vi "Write Plot Data.vi"(10 "Plot Data":cluster{dbl[], dbl[]}[](array[cluster]), 11 "MCCW ACLR in":refnum<class "MCCW ACLR.lvclass">) -> (3 "MCCW ACLR out":refnum<class "MCCW ACLR.lvclass">)   [LabVIEW 2020, in "MCCW ACLR.lvclass"]
uses:
  MCCW ACLR.lvclass
  MCCW ACLR.lvclass/MCCW ACLR.ctl
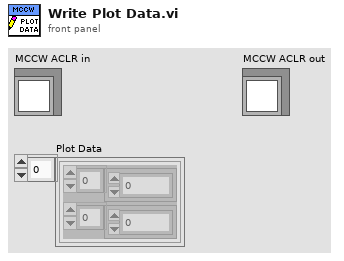
[diagram p1: front panel]
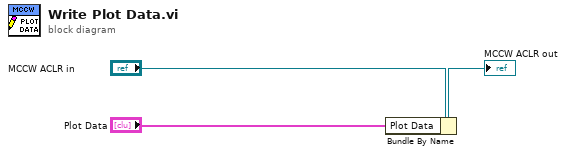
[diagram p0: block diagram]
diagram:
  n1 = Bundle By Name(cluster="MCCW ACLR in", "Plot Data"="Plot Data") -> (→"MCCW ACLR out":refnum<class "MCCW ACLR.lvclass">)
